vi "SetFunctionSampleRate.vi"(8 "error in (no error)":errorcluster, 10 "Variant":variant, 11 "ArbitraryFunction in":refnum<class "ArbitraryFunction.lvclass">) -> (0 "error out":errorcluster, 3 "ArbitraryFunction out":refnum<class "ArbitraryFunction.lvclass">)   [LabVIEW 2018, in "Functions.lvlib" / "ArbitraryFunction.lvclass"]
uses:
  ArbitraryFunction.lvclass
  ArbitraryFunction.lvclass/ArbitraryFunction.ctl
  Accessors/Write SampleRate.vi
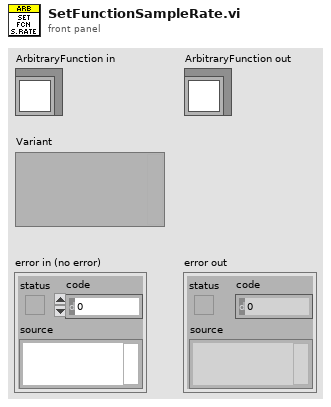
[diagram p1: front panel]
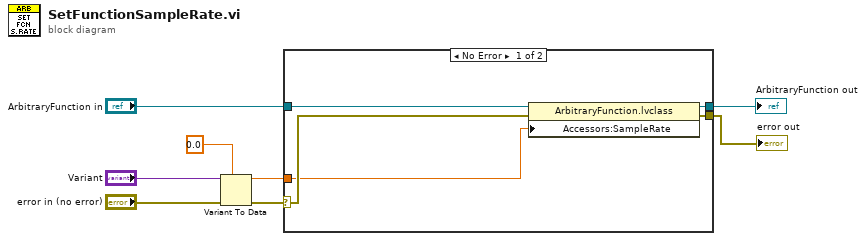
[diagram p0: block diagram]
diagram:
  n1 = Variant To Data(error in="error in (no error)", type=0.0, Variant="Variant") -> (data=w7:dbl, error out=w6:errorcluster)
  n2 = case shown="No Error" w6 {
    selector: w6 -> [w12 w14]
    tunnel: w7 -> [w9 _]
    tunnel: "ArbitraryFunction in" -> [w13 w15]
    tunnel: [w11 w14] -> w4
    tunnel: [w10 w15] -> w5
    frame No Error {
      n3 = property class="ArbitraryFunction.lvclass"(reference=w13, error in=w12, "Accessors:SampleRate"=w9) -> (reference out=w10:refnum<class "ArbitraryFunction.lvclass">, error out=w11:errorcluster)
    }
    frame Error {
    }
  }
  "error out" <- w4
  "ArbitraryFunction out" <- w5
